vi "Read Limit Test Result.vi"(8 "error in (no error)":errorcluster, 9 "Maximum Time (120000 ms)":i32=120000, 10 "Limit Line Number (1: Line1)":i32(ring)=1 items=["Line1"=1, "Line2"=2], 11 "VISA resource name":refnum<visa-resource-name>) -> (0 "error out":errorcluster, 2 "Limit Test Result":dbl, 3 "VISA resource name out":refnum<visa-resource-name>)   [LabVIEW 2022 SP3, in "Agilent N934X Series.lvlib"]
doc: "Read the limits pass/failed result."
uses:
  <instrlib>/Agilent N934X Series/Agilent N934X Series.lvlib
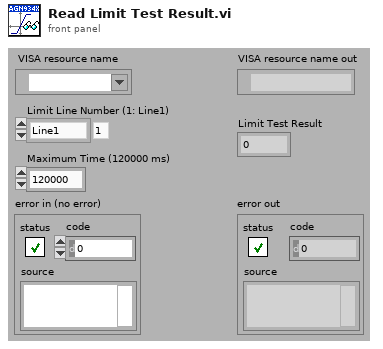
[diagram p1: front panel]
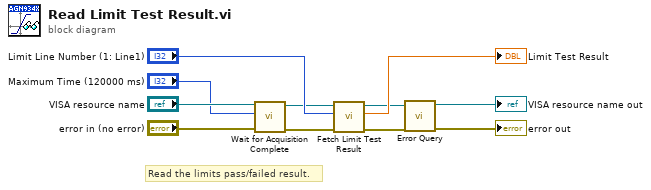
[diagram p0: block diagram]
diagram:
  # "Read the limits pass/failed result."
  n1 = call <instrlib>:"Wait for Acquisition Complete.vi"("error in (no error)"="error in (no error)", "Maximum Time (10000 ms)"="Maximum Time (120000 ms)", "VISA resource name"="VISA resource name") -> ("error out"=w3:errorcluster, "VISA resource name out"=w4:refnum<visa-resource-name>)  [unwired: 7 in]
  n2 = call <instrlib>:"Fetch Limit Test Result.vi"("error in (no error)"=w3, "Limit Line Number (1: Line 1)"="Limit Line Number (1: Line1)", "VISA resource name"=w4) -> ("error out"=w8:errorcluster, "Limit Test Result"=→"Limit Test Result":dbl, "VISA resource name out"=w9:refnum<visa-resource-name>)  [unwired: 6 in]
  n3 = call <instrlib>:"Error Query.vi"("error in (no error)"=w8, "VISA resource name"=w9) -> ("error out"=→"error out":errorcluster, "VISA resource name out"=→"VISA resource name out":refnum<visa-resource-name>)  [unwired: 6 in, 2 out]
